vi "Strip CSM name.vi"(8 "error in":errorcluster, 11 "CSM name":string) -> (0 "error out":errorcluster, 1 "CSM name suffix":string, 2 "matched name part":string, 3 "CSM name core":string)   [LabVIEW 2017, in "CSM-Testcase.lvlib"]
uses:
  CSM-Testcase.lvlib
  src/user.lib/_NEVSTOP/Communicable State Machine(CSM)/_Support/Error/CSM Invalid Name Error.vi
  src/user.lib/_NEVSTOP/Communicable State Machine(CSM)/Communicable State Machine.lvlib
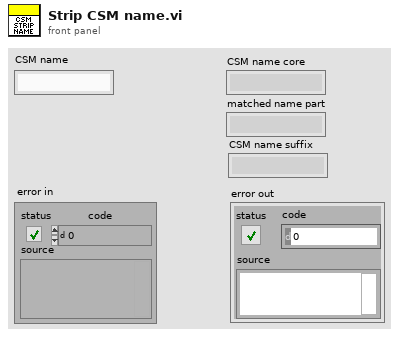
[diagram p1: front panel]
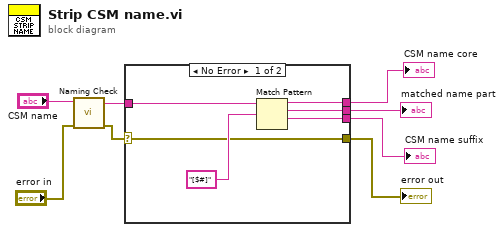
[diagram p0: block diagram]
diagram:
  n1 = call "Naming Check.vi"("error in (no error)"="error in", "Name (\"\" to Use UUID)"="CSM name") -> ("error out"=w5:errorcluster, "Name (Dup)"=w7:string)  [unwired: 8 in]
  n2 = case shown="No Error" w5 {
    selector: w5 -> [w11 w15]
    tunnel: w7 -> [w14 _]
    tunnel: [w11 w15] -> w1
    tunnel: [w12 _] -> w4
    tunnel: [w10 _] -> w3
    tunnel: [w9 _] -> w2
    frame No Error {
      n3 = Match Pattern(string=w14, regular expression="[$#]") -> (before substring=w12:string, match substring=w10:string, after substring=w9:string)  [unwired: 1 in, 1 out]
    }
    frame Error {
    }
  }
  "CSM name core" <- w4
  "matched name part" <- w3
  "CSM name suffix" <- w2
  "error out" <- w1
